vi "set_plot_scale_lc.vi"(8 "set_scale":bool, 9 "lc_scale_settings":enum32{"autoscale", "fancy_scale", "zero_scale"}(ring), 11 "plot_lc_ref":refnum<vi>) -> ()   [LabVIEW 2025]
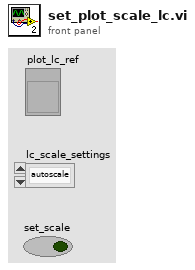
[diagram p1: front panel]
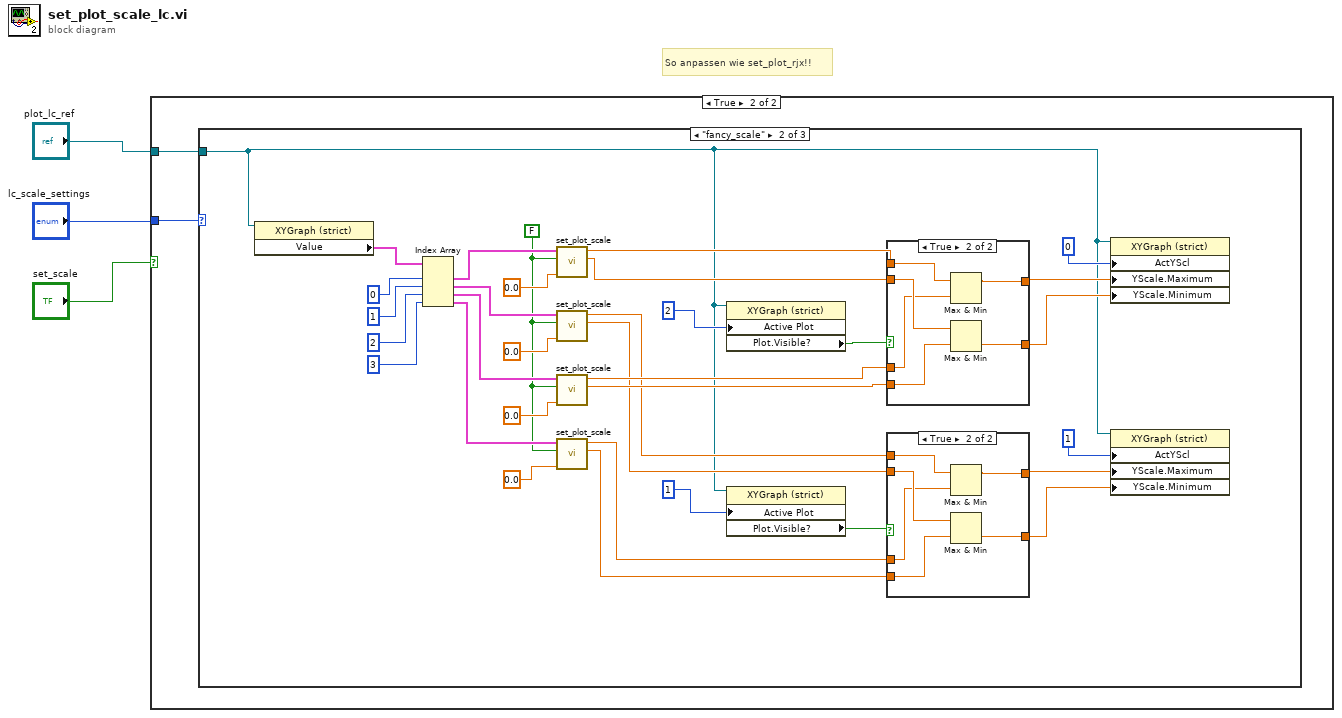
[diagram p0: block diagram]
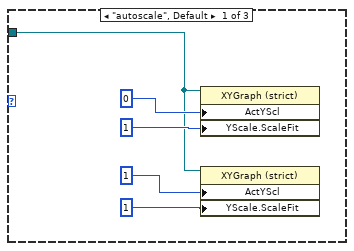
[diagram p3: hidden frame]
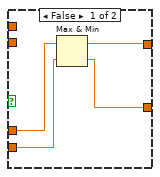
[diagram p4: hidden frame]
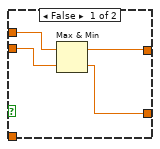
[diagram p5: hidden frame]
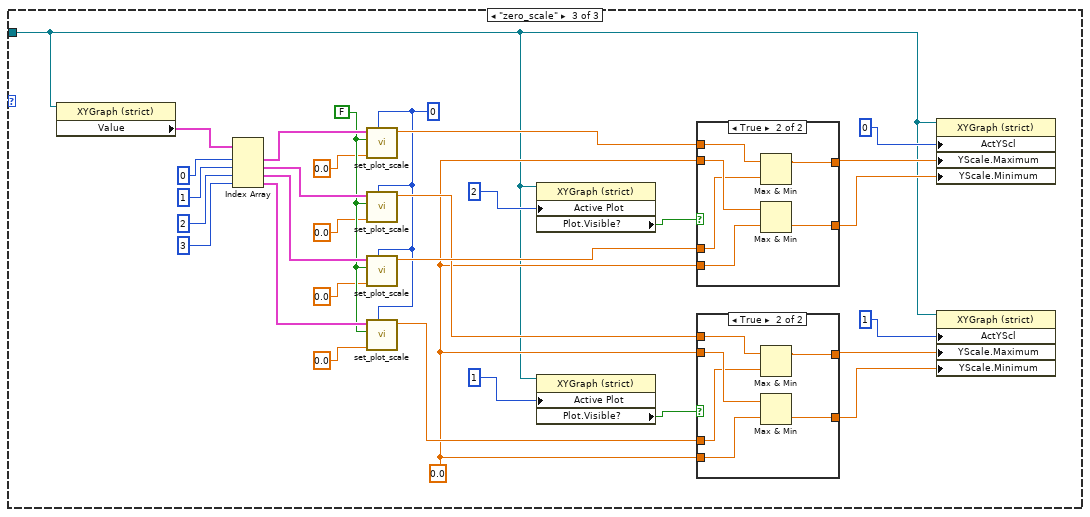
[diagram p6: hidden frame]
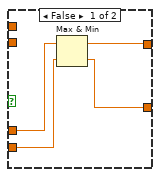
[diagram p7: hidden frame]
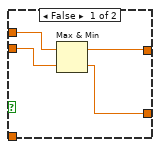
[diagram p8: hidden frame]
diagram:
  # "So anpassen wie set_plot_rjx!!"
  n1 = case shown="True" "set_scale" {
    tunnel: "lc_scale_settings" -> [_ w5]
    tunnel: "plot_lc_ref" -> [_ w4]
    frame False {
    }
    frame True {
      n2 = case shown="\"fancy_scale\"" w5 {
        tunnel: w4 -> [w6 w11 w65]
        frame "autoscale", Default {
          n3 = property on="Property Node" class="XYGraph (strict)"(reference=w6, "ActYScl"=0 ("Active Y Scale"), "YScale.ScaleFit"=u8 1 ("Y Scale.Scale Fit")) -> ()  [unwired: 1 in, 2 out]
          n4 = property on="Property Node" class="XYGraph (strict)"(reference=w6, "ActYScl"=1 ("Active Y Scale"), "YScale.ScaleFit"=u8 1 ("Y Scale.Scale Fit")) -> ()  [unwired: 1 in, 2 out]
        }
        frame "fancy_scale" {
          w23 = FALSE ("round")
          n5 = property on="Property Node" class="XYGraph (strict)"(reference=w11) -> ("Value"=w18:cluster{"array type (2D Dbl)":dbl[], dbl[]}[])  [unwired: 1 in, 2 out]
          n6 = Index Array(array=w18, index #1=0 ("index"), index #2=1 ("index"), index #3=2 ("index"), index #4=3 ("index")) -> (element #1=w42:cluster{"array type (2D Dbl)":dbl[], dbl[]}, element #2=w40:cluster{"array type (2D Dbl)":dbl[], dbl[]}, element #3=w38:cluster{"array type (2D Dbl)":dbl[], dbl[]}, element #4=w36:cluster{"array type (2D Dbl)":dbl[], dbl[]})
          n7 = call "set_plot_scale.vi"("offset"=0.0 ("x"), "round"=w23, "plot_data"=w42) -> ("y_min"=w33:dbl, "y_max"=w34:dbl)  [unwired: 7 in]
          n8 = call "set_plot_scale.vi"("offset"=0.0 ("x"), "round"=w23, "plot_data"=w40) -> ("y_min"=w30:dbl, "y_max"=w31:dbl)  [unwired: 7 in]
          n9 = call "set_plot_scale.vi"("offset"=0.0 ("x"), "round"=w23, "plot_data"=w38) -> ("y_min"=w35:dbl, "y_max"=w32:dbl)  [unwired: 7 in]
          n10 = call "set_plot_scale.vi"("offset"=0.0 ("x"), "round"=w23, "plot_data"=w36) -> ("y_min"=w28:dbl, "y_max"=w29:dbl)  [unwired: 7 in]
          n11 = property on="Property Node" class="XYGraph (strict)"(reference=w11, "Active Plot"=u32 2) -> ("Plot.Visible?"=w21:bool)  [unwired: 1 in, 2 out]
          n12 = property on="Property Node" class="XYGraph (strict)"(reference=w11, "Active Plot"=u32 1) -> ("Plot.Visible?"=w22:bool)  [unwired: 1 in, 2 out]
          n13 = case shown="True" w21 {
            tunnel: w33 -> [w56 w61]
            tunnel: [w54 w63] -> w16
            tunnel: [w55 w62] -> w17
            tunnel: w34 -> [w57 w60]
            tunnel: w32 -> [_ w59]
            tunnel: w35 -> [_ w58]
            frame False {
              n14 = Max & Min(x=w57, y=w56) -> (max(x,y)=w54:dbl, min(x,y)=w55:dbl)
            }
            frame True {
              n15 = Max & Min(x=w60, y=w59) -> (max(x,y)=w63:dbl)  [unwired: 1 out]
              n16 = Max & Min(x=w61, y=w58) -> (min(x,y)=w62:dbl)  [unwired: 1 out]
            }
          }
          n17 = case shown="True" w22 {
            tunnel: w30 -> [_ w51]
            tunnel: [w46 w53] -> w13
            tunnel: [w47 w52] -> w12
            tunnel: w31 -> [_ w50]
            tunnel: w29 -> [w44 w49]
            tunnel: w28 -> [w45 w48]
            frame False {
              n18 = Max & Min(x=w44, y=w45) -> (max(x,y)=w46:dbl, min(x,y)=w47:dbl)
            }
            frame True {
              n19 = Max & Min(x=w50, y=w49) -> (max(x,y)=w53:dbl)  [unwired: 1 out]
              n20 = Max & Min(x=w51, y=w48) -> (min(x,y)=w52:dbl)  [unwired: 1 out]
            }
          }
          n21 = property on="Property Node" class="XYGraph (strict)"(reference=w11, "ActYScl"=0 ("Active Y Scale"), "YScale.Maximum"=w16, "YScale.Minimum"=w17) -> ()  [unwired: 1 in, 2 out]
          n22 = property on="Property Node" class="XYGraph (strict)"(reference=w11, "ActYScl"=1 ("Active Y Scale"), "YScale.Maximum"=w13, "YScale.Minimum"=w12) -> ()  [unwired: 1 in, 2 out]
        }
        frame "zero_scale" {
          w64 = 0 ("pos_neg_both")
          w78 = 0.0 ("y_min")
          w86 = FALSE ("round")
          n23 = property on="Property Node" class="XYGraph (strict)"(reference=w65) -> ("Value"=w76:cluster{"array type (2D Dbl)":dbl[], dbl[]}[])  [unwired: 1 in, 2 out]
          n24 = Index Array(array=w76, index #1=0 ("index"), index #2=1 ("index"), index #3=2 ("index"), index #4=3 ("index")) -> (element #1=w94:cluster{"array type (2D Dbl)":dbl[], dbl[]}, element #2=w93:cluster{"array type (2D Dbl)":dbl[], dbl[]}, element #3=w92:cluster{"array type (2D Dbl)":dbl[], dbl[]}, element #4=w91:cluster{"array type (2D Dbl)":dbl[], dbl[]})
          n25 = call "set_plot_scale.vi"("pos_neg_both"=w64, "offset"=0.0 ("x"), "round"=w86, "plot_data"=w94) -> ("y_max"=w77:dbl)  [unwired: 6 in, 1 out]
          n26 = call "set_plot_scale.vi"("pos_neg_both"=w64, "offset"=0.0 ("x"), "round"=w86, "plot_data"=w93) -> ("y_max"=w89:dbl)  [unwired: 6 in, 1 out]
          n27 = call "set_plot_scale.vi"("pos_neg_both"=w64, "offset"=0.0 ("x"), "round"=w86, "plot_data"=w92) -> ("y_max"=w90:dbl)  [unwired: 6 in, 1 out]
          n28 = call "set_plot_scale.vi"("pos_neg_both"=w64, "offset"=0.0 ("x"), "round"=w86, "plot_data"=w91) -> ("y_max"=w88:dbl)  [unwired: 6 in, 1 out]
          n29 = property on="Property Node" class="XYGraph (strict)"(reference=w65, "Active Plot"=u32 2) -> ("Plot.Visible?"=w74:bool)  [unwired: 1 in, 2 out]
          n30 = property on="Property Node" class="XYGraph (strict)"(reference=w65, "Active Plot"=u32 1) -> ("Plot.Visible?"=w75:bool)  [unwired: 1 in, 2 out]
          n31 = case shown="True" w74 {
            tunnel: w78 -> [w107 w112]
            tunnel: [w105 w114] -> w67
            tunnel: [w106 w113] -> w66
            tunnel: w77 -> [w108 w111]
            tunnel: w90 -> [_ w110]
            tunnel: w78 -> [_ w109]
            frame False {
              n32 = Max & Min(x=w108, y=w107) -> (max(x,y)=w105:dbl, min(x,y)=w106:dbl)
            }
            frame True {
              n33 = Max & Min(x=w111, y=w110) -> (max(x,y)=w114:dbl)  [unwired: 1 out]
              n34 = Max & Min(x=w112, y=w109) -> (min(x,y)=w113:dbl)  [unwired: 1 out]
            }
          }
          n35 = case shown="True" w75 {
            tunnel: w78 -> [_ w102]
            tunnel: [w97 w104] -> w70
            tunnel: [w98 w103] -> w69
            tunnel: w89 -> [_ w101]
            tunnel: w88 -> [w95 w100]
            tunnel: w78 -> [w96 w99]
            frame False {
              n36 = Max & Min(x=w95, y=w96) -> (max(x,y)=w97:dbl, min(x,y)=w98:dbl)
            }
            frame True {
              n37 = Max & Min(x=w101, y=w100) -> (max(x,y)=w104:dbl)  [unwired: 1 out]
              n38 = Max & Min(x=w102, y=w99) -> (min(x,y)=w103:dbl)  [unwired: 1 out]
            }
          }
          n39 = property on="Property Node" class="XYGraph (strict)"(reference=w65, "ActYScl"=0 ("Active Y Scale"), "YScale.Maximum"=w67, "YScale.Minimum"=w66) -> ()  [unwired: 1 in, 2 out]
          n40 = property on="Property Node" class="XYGraph (strict)"(reference=w65, "ActYScl"=1 ("Active Y Scale"), "YScale.Maximum"=w70, "YScale.Minimum"=w69) -> ()  [unwired: 1 in, 2 out]
        }
      }
    }
  }
